vi "Periodic Tasks.vi"(8 "error in":errorcluster) -> ()   [LabVIEW 2018]
doc: "This VI runs in parallel to other tasks. It can contain as many user-defined periodic loops as you need. These can carry out PID or other sorts of timed response."
uses:
  <vilib>/Analysis/coordinate.llb/Angle Units.ctl
  <vilib>/Analysis/coordinate.llb/Angle Range (Degree).ctl
  <vilib>/Analysis/coordinate.llb/Wrap Angle (scalar).vi
  <vilib>/Rock Robotics/WPI/Utilities/WPI_GetSetVariantRefNum.vi
  Robot Global Data.vi
  <vilib>/Analysis/NI_AAL_Angle.lvlib
panel:
  out "Front Right Encoder":dbl=509.0
  out "Back Right Encoder":dbl=36.0
  out "Back Left Encoder":dbl
  out "Front Left Encoder":dbl
  in  "Back Right Offset":dbl=37.0
  in  "Front Right Offset":dbl=512.0
  out "Back Right Angle":dbl
  out "Front Right Angle":dbl
  in  "Back Left Offset":dbl=19.0
  in  "Front Left Offset":dbl=188.0
  out "Back Left Angle":dbl
  out "Front Left Angle":dbl
  # "Click here to set min"
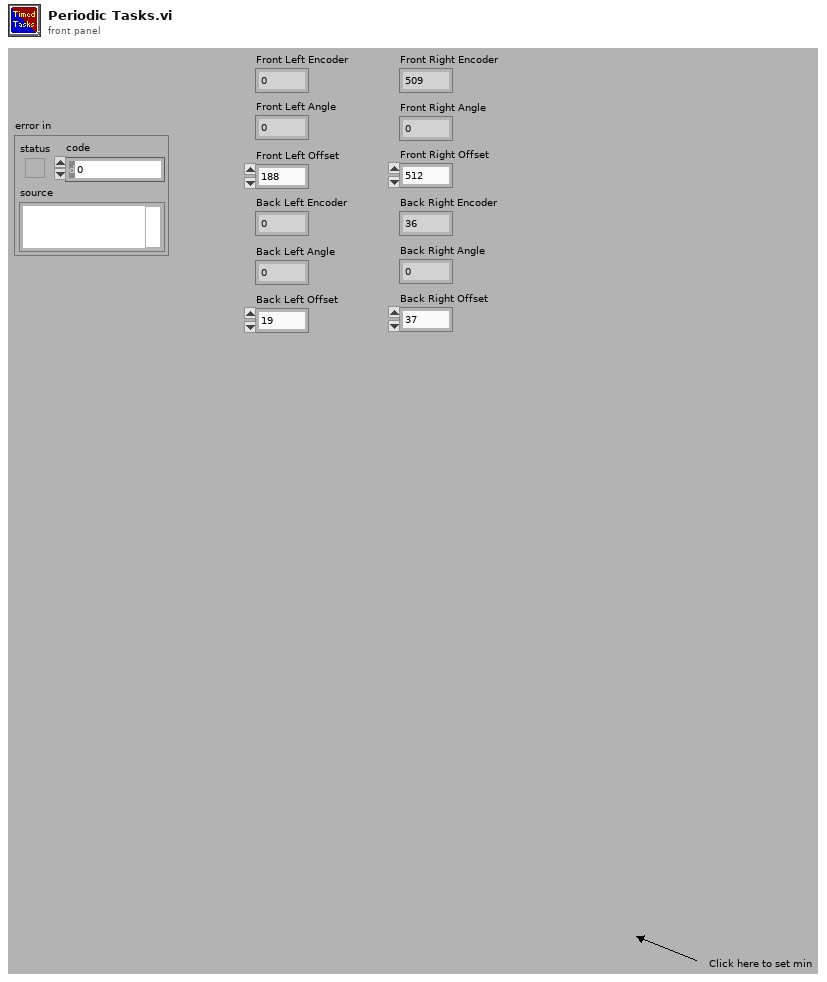
[diagram p1: front panel]
types:
  T1 = typedef "WPI_RobotDriveDevRef.ctl" = cluster{"DevStatus":errorcluster, "Motors[]":T2[], "Square Inputs":bool, "Max Output":dbl}
  T2 = typedef "WPI_MotorControlDeviceRef.ctl" = cluster{"DeviceStatus":errorcluster, "Type":T3, "PWM":cluster{"PWM Channel":T4, "DeadBand":T5}, "CAN":cluster{"Device Number":u8, "SetOutput VI Ref":variant, "GetOutput VI Ref":variant, "Enable VI Ref":variant, "Disable VI Ref":variant, "Data":variant}, "Invert":bool, "DIO PWM":cluster{"PWM \"Enable\" Channel":T4, "DIOChannel":T6, "PWM Rate":dbl}}
  T3 = typedef "WPI_MotorControlType.ctl" = enum16{"PWM", "CAN", "DIO PWM"}
  T4 = typedef "FPGA_DIOPWMChannel.ctl" = enum8{"PWM 0", "PWM 1", "PWM 2", "PWM 3", "PWM 4", "PWM 5", "PWM 6", "PWM 7", "PWM 8", "PWM 9", "PWM MXP 0", "PWM MXP 1", "PWM MXP 2", "PWM MXP 3", "PWM MXP 4", "PWM MXP 5", "PWM MXP 6", "PWM MXP 7", "PWM MXP 8", "PWM MXP 9", "Invalid"}
  T5 = typedef "WPI_PWMDeadband.ctl" = cluster{"Name":string, "maxPositivePwm":i32, "minPositivePwm":i32, "centerPwm":i32, "maxNegativePwm":i32, "minNegativePwm":i32, "angularRange":u16}
  T6 = typedef "FPGA_DIOChannel.ctl" = enum8{"DIO 0", "DIO 1", "DIO 2", "DIO 3", "DIO 4", "DIO 5", "DIO 6", "DIO 7", "DIO 8", "DIO 9", "DIO MXP 0", "DIO MXP 1", "DIO MXP 2", "DIO MXP 3", "DIO MXP 4", "DIO MXP 5", "DIO MXP 6", "DIO MXP 7", "DIO MXP 8", "DIO MXP 9", "DIO MXP 10", "DIO MXP 11", "DIO MXP 12", "DIO MXP 13", "DIO MXP 14", "DIO MXP 15", "SPI Port CS1", "SPI Port CS2", "SPI Port CS3", "SPI Port MISO", "SPI Port MOSI", "Invalid"}
  T7 = typedef "WPI_JoystickDevRef.ctl" = cluster{"Device":T8}
  T8 = typedef "WPI_JoystickDeviceEnum.ctl" = enum16{"USB 0", "USB 1", "USB 2", "USB 3", "USB 4", "USB 5"}
  T9 = cluster{"JoystickDevRef":T7, "RobotDriveDevRef":T1}
  T10 = typedef "NI_AAL_Angle.lvlib/Angle Range (Degree).ctl" = u16
  T11 = typedef "NI_AAL_Angle.lvlib/Angle Units.ctl" = i32
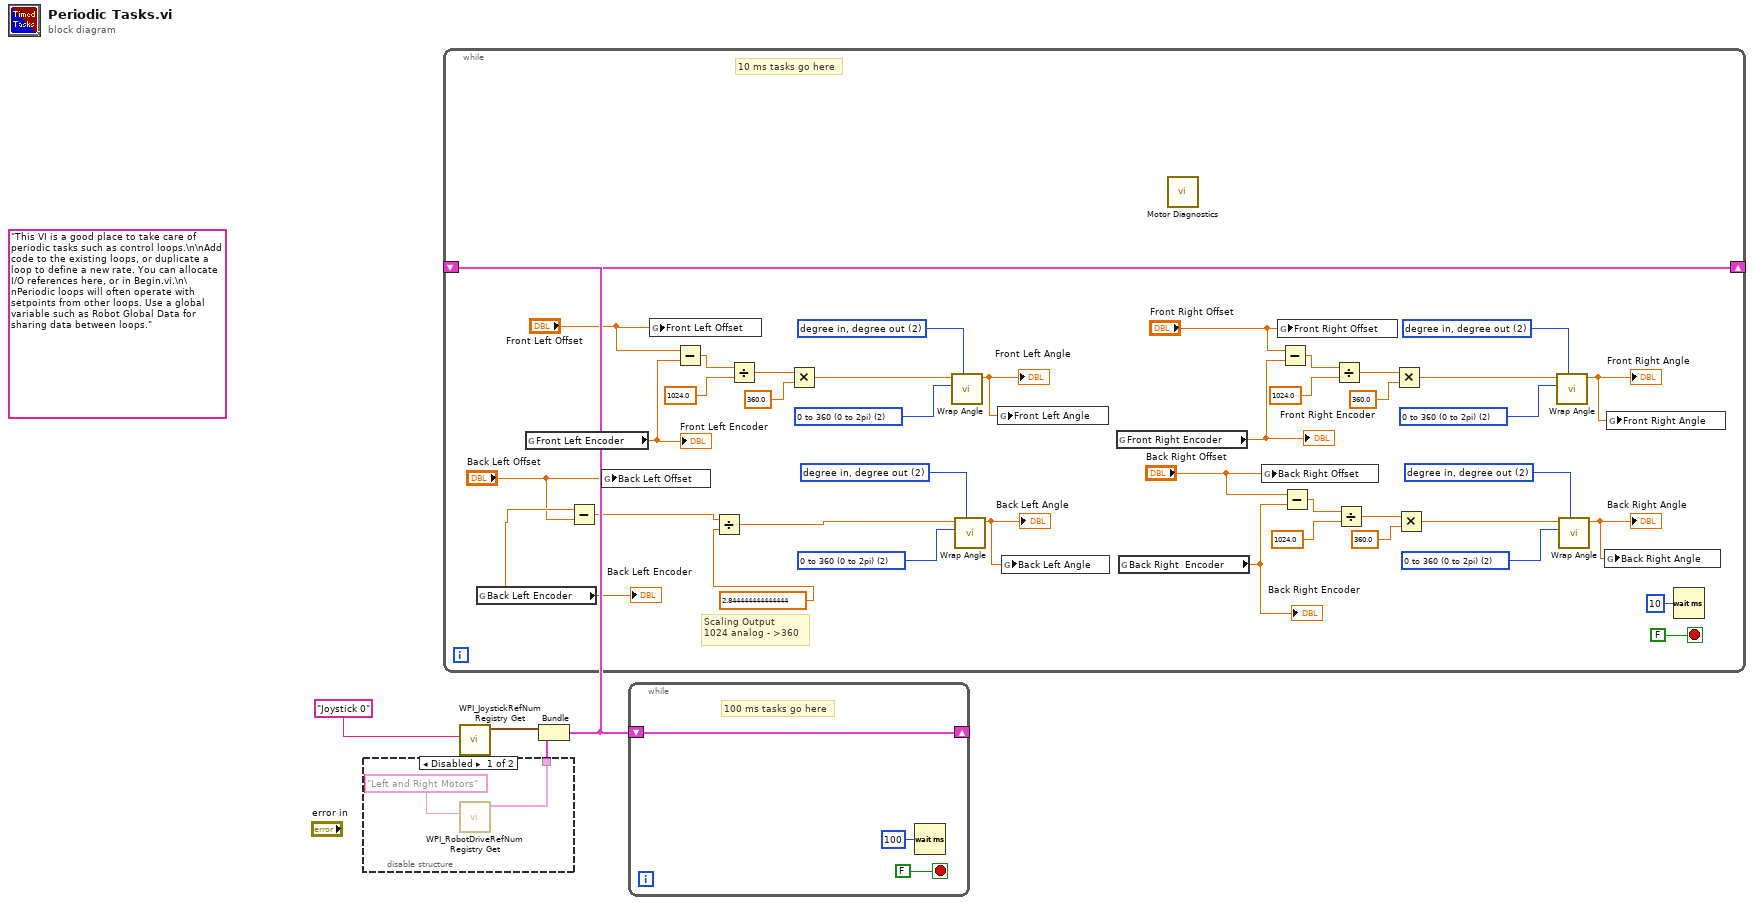
[diagram p0: block diagram]
diagram:
  (unwired) "This VI is a good place to take care of periodic tasks such as control loops.\n\nAdd code to the existing loops, or duplicate a loop to define a new rate. You can allocate I/O references here, or in Begin.vi.\n\nPeriodic loops will often operate with setpoints from other loops. Use a global variable such as Robot Global Data for sharing data between loops."
  n1 = disable-structure shown="Disabled" {
    disable-tunnel: [w5 _] -> w2
    frame Disabled {
      n2 = call <vilib>:"WPI_RobotDriveRefNum Registry Get.vi"("refnum name"="Left and Right Motors") -> ("RobotDriveDevRef"=w5:T1)  [unwired: 1 in, 9 out]
    }
    frame Enabled {
    }
  }
  n3 = call <vilib>:"WPI_JoystickRefNum Registry Get.vi"("refnum name"="Joystick 0") -> ("JoystickDevRef"=w3:T7)  [unwired: 1 in, 9 out]
  n4 = Bundle("JoystickDevRef"=w3, "RobotDriveDevRef"=w2) -> (w1:T9)  [unwired: 1 out]
  n5 = while {
    shift-right: [w45] -> _
    shift-left: w1 -> [w45]
    stop <- FALSE stop-if-true
    w20 = T10 2 items=["none", "-180 to 180 (-pi to pi)", "0 to 360 (0 to 2pi)"] ("angle range")
    w21 = T11 2 items=["radian in, radian out", "radian in, degree out", "degree in, degree out", "degree in, radian out"] ("angle units")
    w24 = T10 2 items=["none", "-180 to 180 (-pi to pi)", "0 to 360 (0 to 2pi)"] ("angle range")
    w25 = T11 2 items=["radian in, radian out", "radian in, degree out", "degree in, degree out", "degree in, radian out"] ("angle units")
    w33 = T10 2 items=["none", "-180 to 180 (-pi to pi)", "0 to 360 (0 to 2pi)"] ("angle range")
    w34 = T11 2 items=["radian in, radian out", "radian in, degree out", "degree in, degree out", "degree in, radian out"] ("angle units")
    w40 = T10 2 items=["none", "-180 to 180 (-pi to pi)", "0 to 360 (0 to 2pi)"] ("angle range")
    w41 = T11 2 items=["radian in, radian out", "radian in, degree out", "degree in, degree out", "degree in, radian out"] ("angle units")
    # "Scaling Output\n1024 analog - >360"
    # "10 ms tasks go here"
    n6 = global read "Robot Global Data.vi" "Back Left Encoder"() -> (w8:dbl)
    "Back Left Encoder" <- w8
    n7 = global read "Robot Global Data.vi" "Front Left Encoder"() -> (w13:dbl)
    "Front Left Encoder" <- w13
    n8 = Subtract(x=w8, y="Back Left Offset") -> (x-y=w11:dbl)
    n9 = global write "Robot Global Data.vi" "Back Left Offset"("Back Left Offset") -> ()
    n10 = global write "Robot Global Data.vi" "Front Left Offset"("Front Left Offset") -> ()
    n11 = Subtract(x="Front Left Offset", y=w13) -> (x-y=w27:dbl)
    n12 = Divide(x=w11, y=2.844444444444444) -> (x/y=w9:dbl)
    n13 = Divide(x=w27, y=1024.0 ("x")) -> (x/y=w23:dbl)
    n14 = Multiply(x=w23, y=360.0 ("x*y")) -> (x*y=w22:dbl)
    n15 = call-poly <vilib>:"Wrap Angle.vi"("angle units"=w25, "angle range"=w24, "angle in"=w22) -> ("angle out"=w19:dbl)  [unwired: 7 in, 1 out]
    "Front Left Angle" <- w19
    n16 = call-poly <vilib>:"Wrap Angle.vi"("angle units"=w21, "angle range"=w20, "angle in"=w9) -> ("angle out"=w18:dbl)  [unwired: 7 in, 1 out]
    "Back Left Angle" <- w18
    n17 = global write "Robot Global Data.vi" "Front Left Angle"(w19) -> ()
    n18 = global write "Robot Global Data.vi" "Back Left Angle"(w18) -> ()
    n19 = global read "Robot Global Data.vi" "Front Right Encoder"() -> (w17:dbl)
    "Front Right Encoder" <- w17
    n20 = global read "Robot Global Data.vi" "Back Right  Encoder"() -> (w16:dbl)
    "Back Right Encoder" <- w16
    n21 = call "Motor Diagnostics.vi"() -> ()  [unwired: 2 in]
    n22 = global write "Robot Global Data.vi" "Back Right Offset"("Back Right Offset") -> ()
    n23 = global write "Robot Global Data.vi" "Front Right Offset"("Front Right Offset") -> ()
    n24 = Subtract(x="Front Right Offset", y=w17) -> (x-y=w43:dbl)
    n25 = Subtract(x="Back Right Offset", y=w16) -> (x-y=w36:dbl)
    n26 = Divide(x=w43, y=1024.0 ("x")) -> (x/y=w39:dbl)
    n27 = Divide(x=w36, y=1024.0 ("x")) -> (x/y=w32:dbl)
    n28 = Multiply(x=w39, y=360.0 ("x*y")) -> (x*y=w38:dbl)
    n29 = Multiply(x=w32, y=360.0 ("x*y")) -> (x*y=w31:dbl)
    n30 = call-poly <vilib>:"Wrap Angle.vi"("angle units"=w41, "angle range"=w40, "angle in"=w38) -> ("angle out"=w30:dbl)  [unwired: 7 in, 1 out]
    "Front Right Angle" <- w30
    n31 = call-poly <vilib>:"Wrap Angle.vi"("angle units"=w34, "angle range"=w33, "angle in"=w31) -> ("angle out"=w29:dbl)  [unwired: 7 in, 1 out]
    "Back Right Angle" <- w29
    n32 = global write "Robot Global Data.vi" "Back Right Angle"(w29) -> ()
    n33 = global write "Robot Global Data.vi" "Front Right Angle"(w30) -> ()
    n34 = Wait (ms)(milliseconds to wait=u32 10) -> ()  [unwired: 1 out]
  }
  n35 = while {
    shift-right: [w48] -> _
    shift-left: w1 -> [w48]
    stop <- FALSE stop-if-true
    # "100 ms tasks go here"
    n36 = Wait (ms)(milliseconds to wait=u32 100) -> ()  [unwired: 1 out]
  }
